vi "magnitude_dbl.vi"(4 "vector":dbl[](array[numeric])) -> (1 "vector magnitude":dbl)   [LabVIEW 2013]
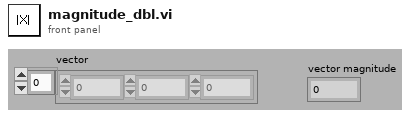
[diagram p1: front panel]
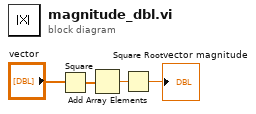
[diagram p0: block diagram]
diagram:
  n1 = Square(x="vector") -> (x^2=w4:dbl[])
  n2 = Add Array Elements(numeric array=w4) -> (sum=w3:dbl)
  n3 = Square Root(x=w3) -> (sqrt(x)=→"vector magnitude":dbl)
